vi "Open Connection_TangentActuatorAbsolutePositionSteps.vi"(8 "error in (no error)":errorcluster, 9 "TangentActuatorAbsolutePositionSteps":T1, 10 "topicName":string) -> (0 "error out":errorcluster, 3 "topicRef":cluster{"topicName":string, "type":refnum<vi>})   [LabVIEW 2015]
uses:
  SALTypedefs/m2ms/TangentActuatorAbsolutePositionSteps.ctl
  SALTypedefs/m2ms/m2ms.lvlib
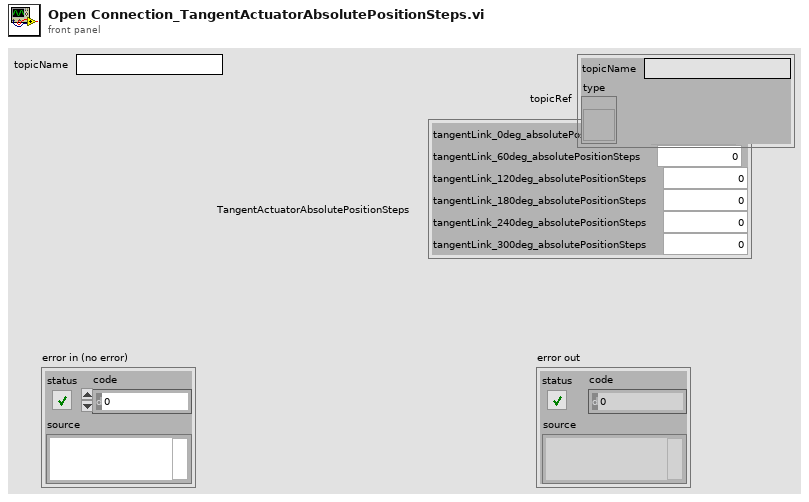
[diagram p1: front panel]
types:
  T1 = typedef "m2ms.lvlib/TangentActuatorAbsolutePositionSteps.ctl" = cluster{"tangentLink_0deg_absolutePositionSteps":i32, "tangentLink_60deg_absolutePositionSteps":i32, "tangentLink_120deg_absolutePositionSteps":i32, "tangentLink_180deg_absolutePositionSteps":i32, "tangentLink_240deg_absolutePositionSteps":i32, "tangentLink_300deg_absolutePositionSteps":i32}
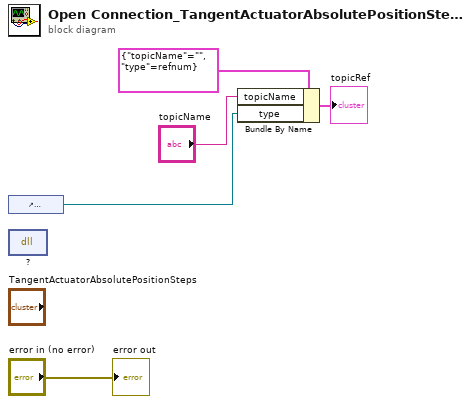
[diagram p0: block diagram]
diagram:
  n1 = control-ref of="TangentActuatorAbsolutePositionSteps"() -> (w2:refnum<vi>)
  n2 = dll-call lib="?" fn="?"() -> ()  [unwired: 4 in, 2 out]
  n3 = Bundle By Name(cluster=cluster{"topicName":string, "type":refnum<vi>} {"topicName"="", "type"=refnum} ("topicRef"), "topicName"="topicName", "type"=w2) -> (→"topicRef":cluster{"topicName":string, "type":refnum<vi>})
  "error out" <- "error in (no error)"
